vi "FTW-SEQ-Destroy.vi"(1 "Sequencer":refnum<class "FTW-Sequencer.lvclass">) -> ()   [LabVIEW 2012, in "FTW-Sequencer.lvclass"]
uses:
  FTW-Sequencer.lvclass
panel:
  # "Inputs"
  # "Outputs"
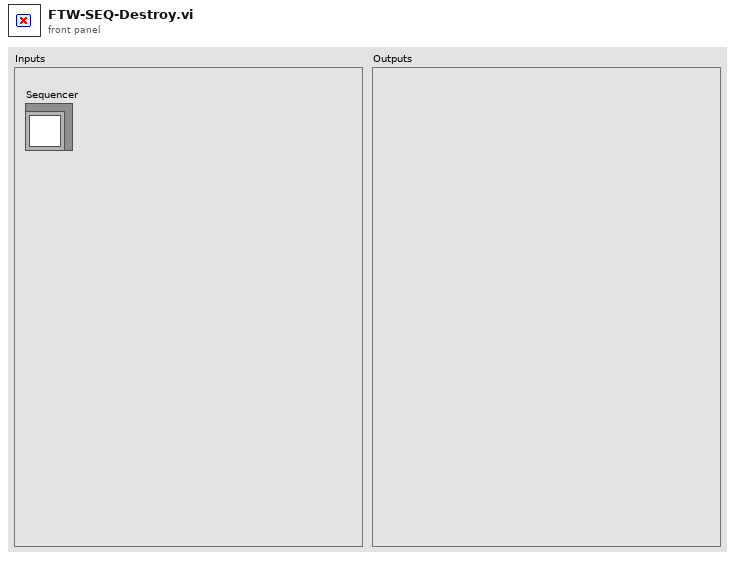
[diagram p1: front panel]
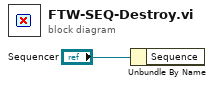
[diagram p0: block diagram]
diagram:
  n1 = Unbundle By Name("Sequencer") -> ()  [unwired: 1 out]
